vi "Circular Buffer Array LV2012 NIVerified.vi"() -> ()   [LabVIEW 2016]
panel:
  out "Circular Array":i32[](array[numeric])
  in  "Array Size":i32=10
  in  "stop":bool
  # "Overview: Create a user-defined circular buffer\nRequirements: LabVIEW 2012 (or compatible)\nInstructions: \nSpecify the size of the array\nRun the code"
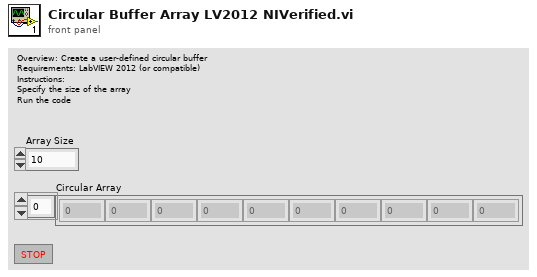
[diagram p1: front panel]
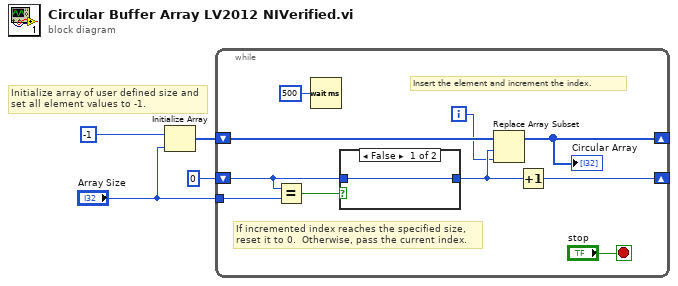
[diagram p0: block diagram]
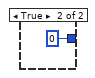
[diagram p2: hidden frame]
diagram:
  # "Initialize array of user defined size and set all element values to -1."
  n1 = Initialize Array(-1, "Array Size") -> (w4:i32[])
  n2 = while {
    shift-right: [w10] -> _
    shift-left: 0 -> [w13]
    shift-right: [w8] -> _
    shift-left: w4 -> [w12]
    tunnel: "Array Size" -> [w7]
    i -> [w6]
    stop <- "stop" stop-if-true
    # "If incremented index reaches the specified size, reset it to 0.  Otherwise, pass the current index."
    # "Insert the element and increment the index."
    n3 = Equal?(x=w13, y=w7) -> (x = y?=w14:bool)
    n4 = Wait (ms)(milliseconds to wait=u32 500 ("millisecond multiple")) -> ()  [unwired: 1 out]
    n5 = case shown="False" w14 {
      tunnel: w13 -> [w15 _]
      tunnel: [w15 0] -> w11
      frame False {
      }
      frame True {
      }
    }
    n6 = Replace Array Subset "Replace Array Subset"(array=w12, new element=w6, index=w11) -> (w8:i32[])
    "Circular Array" <- w8
    n7 = Increment(x=w11) -> (x+1=w10:i32)
  }
